vi "TDMS Close Retry.vi"(4 "Release File? (T)":bool=TRUE, 6 "New TDMS File Name (Optional)":string, 7 "TDMS Path":path, 8 "error in (no error)":errorcluster, 9 "Operation (0:open)":T1(ring)=enum."open (read-only)", 11 "TDMS File Ref":refnum<k34>) -> (0 "error out":errorcluster, 3 "TDMS Path Out":path, 5 "Execution Time (ms)":u32)   [LabVIEW 2011]
uses:
  Summitek EXT/OpenG EXT/file/file.llb/Convert File Extension (Path)__ogtk.vi
  Summitek EXT/OpenG EXT/file/file.llb/File Exists - Scalar__ogtk.vi
  Summitek EXT/OpenG EXT/file/file.llb/Strip Path Extension - Path__ogtk.vi
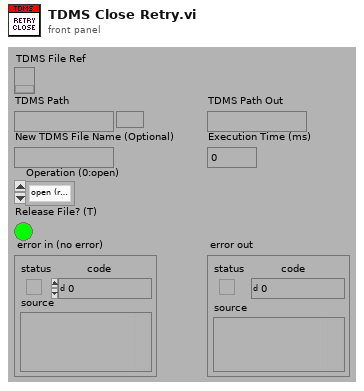
[diagram p1: front panel]
types:
  T1 = enum16{"open", "open or create", "create or replace", "create", "open (read-only)"}
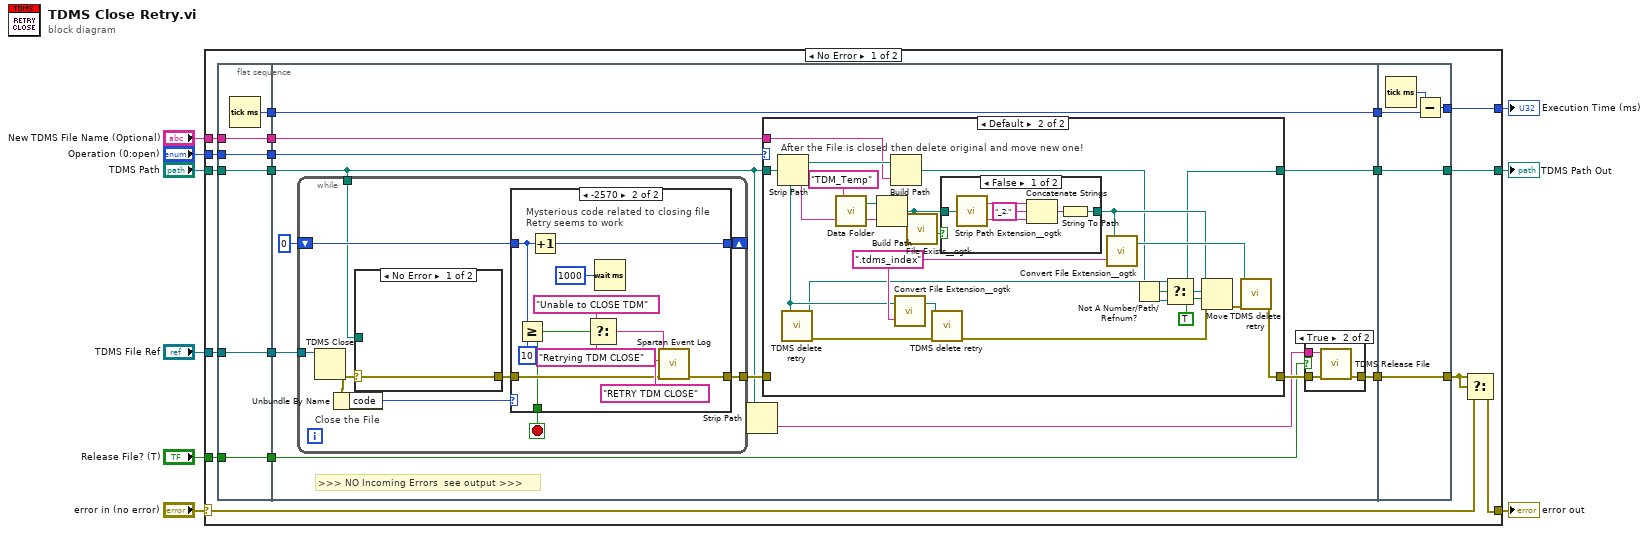
[diagram p0: block diagram]
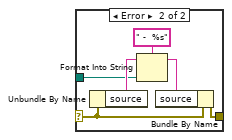
[diagram p5: hidden frame]
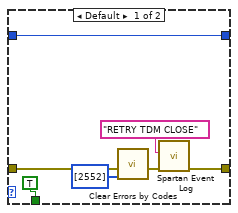
[diagram p6: hidden frame]
diagram:
  n1 = case shown="No Error" "error in (no error)" {
    selector: "error in (no error)" -> [w16 w121]
    tunnel: "TDMS File Ref" -> [w22 _]
    tunnel: "Operation (0:open)" -> [w21 _]
    tunnel: "TDMS Path" -> [w20 w120]
    tunnel: [w19 _] -> w6
    tunnel: [w18 w121] -> w5
    tunnel: [w15 w120] -> w3
    tunnel: "New TDMS File Name (Optional)" -> [w12 _]
    tunnel: "Release File? (T)" -> [w10 _]
    frame No Error {
      n2 = flat-sequence {
        tunnel: w20 -> [w32]
        tunnel: w21 -> [w33]
        tunnel: w22 -> [w34]
        tunnel: [w34] -> w28
        tunnel: [w33] -> w27
        tunnel: [w32] -> w26
        tunnel: [w31] -> w25
        tunnel: [w30] -> w13
        tunnel: w12 -> [w30]
        tunnel: [w29] -> w11
        tunnel: w10 -> [w29]
        tunnel: [w38] -> w24
        tunnel: w28 -> [w45]
        tunnel: w27 -> [w44]
        tunnel: w26 -> [w37]
        tunnel: [w42] -> w23
        tunnel: w25 -> [w42]
        tunnel: [w40] -> w14
        tunnel: w13 -> [w41]
        tunnel: w11 -> [w35]
        tunnel: [w119] -> w17
        tunnel: w24 -> [w119]
        tunnel: w23 -> [w117]
        tunnel: [w116] -> w19
        tunnel: [w115] -> w15
        tunnel: w14 -> [w115]
        frame #0 {
          n3 = Tick Count (ms)() -> (millisecond timer value=w31:u32)
        }
        frame #1 {
          # ">>> NO Incoming Errors  see output >>>"
          n4 = while {
            tunnel: w45 -> [w89]
            shift-right: [w85] -> _
            shift-left: 0 -> [w86]
            tunnel: [w84] -> w43
            tunnel: w37 -> [w81]
            stop <- w88 stop-if-true
            # "Close the File"
            n5 = TDMS Close(11:w89) -> (0:w82:errorcluster)  [unwired: 1 in, 1 out]
            n6 = Unbundle By Name(w82) -> ("code"=w87:i32)
            n7 = case shown="No Error" w82 {
              selector: w82 -> [w90 w93]
              tunnel: w81 -> [_ w94]
              tunnel: [w90 w91] -> w83
              frame No Error {
              }
              frame Error {
                n8 = Unbundle By Name(w93) -> ("source"=w95:string)
                n9 = Format Into String(format string=" -  %s", initial string=w95, w94) -> (resulting string=w92:string)  [unwired: 1 in, 1 out]
                n10 = Bundle By Name(cluster=w93, "source"=w92) -> (w91:errorcluster)
              }
            }
            n11 = case shown="-2570" w87 {
              tunnel: [TRUE ("T button?") w106] -> w88
              tunnel: w83 -> [w98 w113]
              tunnel: w86 -> [w102 w111]
              tunnel: [w102 w112] -> w85
              tunnel: [w101 w105] -> w84
              frame Default {
                n12 = call "Clear Errors by Codes.vi"("Error Codes\nto Clear (Empty)"=i32[] [2552] ("Error Codes\nto Clear (Empty)"), "error in (no error)"=w98) -> ("error out"=w97:errorcluster)  [unwired: 5 out]
                n13 = call "Spartan Event Log.vi"("error in (no error)"=w97, "module (\"\")"="RETRY TDM CLOSE") -> ("error out"=w101:errorcluster)  [unwired: 6 in]
              }
              frame -2570 {
                # "Mysterious code related to closing file\nRetry seems to work"
                n14 = Greater Or Equal?(x=w111, y=10) -> (x >= y?=w106:bool)
                n15 = Increment(x=w111) -> (x+1=w112:i32)
                n16 = Select(t="Unable to CLOSE TDM" ("message (\"\")"), s=w106, f="Retrying TDM CLOSE" ("message (\"\")")) -> (s? t:f=w107:string)
                n17 = Wait (ms)(milliseconds to wait=u32 1000) -> ()  [unwired: 1 out]
                n18 = call "Spartan Event Log.vi"("error in (no error)"=w113, "module (\"\")"="RETRY TDM CLOSE", "message (\"\")"=w107) -> ("error out"=w105:errorcluster)  [unwired: 5 in]
              }
            }
          }
          n19 = Strip Path(path=w37) -> (name=w36:string)  [unwired: 1 out]
          n20 = case shown="Default" w44 {
            tunnel: [w52 w70] -> w39
            tunnel: w43 -> [w52 _]
            tunnel: w37 -> [w51 w60]
            tunnel: w41 -> [_ w58]
            tunnel: [w51 w54] -> w40
            frame "create or replace", "open (read-only)" {
              # "The query TDM use the \"create or replace\" mode for the files.\nThey aren't in the search area.\nRead only operations shouldn't be affected either"
            }
            frame Default {
              w61 = ".tdms_index" ("regular expression")
              # "After the File is closed then delete original and move new one!"
              n21 = Strip Path(path=w60) -> (stripped path=w59:path, name=w73:string)
              n22 = call "TDMS delete retry.vi"("path (use dialog)"=w60) -> ("error out"=w68:errorcluster, "deleted path"=w56:path)  [unwired: 9 out]
              n23 = call "Data Folder.vi"("Relative Path (\"\" - Folder)"="TDM_Temp" ("Relative Path (\"\" - Folder)")) -> ("Data Folder"=w72:path)  [unwired: 2 in]
              n24 = Build Path(base path=w72, name or relative path=w73) -> (appended path=w63:path)
              n25 = Build Path(base path=w59, name or relative path=w58) -> (appended path=w55:path)
              n26 = call-poly "Convert File Extension__ogtk.vi"("new ending (none)"=w61, "file name"=w60) -> ("new filename"=w67:path)  [unwired: 1 out]
              n27 = call-poly "File Exists__ogtk.vi"("file path"=w63) -> ("exists"=w64:bool)  [unwired: 6 in, 1 out]
              n28 = call "TDMS delete retry.vi"("error in"=w68, "path (use dialog)"=w67) -> ("error out"=w71:errorcluster)  [unwired: 9 out]
              n29 = case shown="False" w64 {
                tunnel: w63 -> [w74 w80]
                tunnel: [w75 w80] -> w62
                frame False {
                  n30 = call-poly "Strip Path Extension__ogtk.vi"("path"=w74) -> ("root"=w77:string, "extension"=w76:string)
                  n31 = Concatenate Strings(w77, "_2." ("string"), w76) -> (w79:string)
                  n32 = String To Path(string=w79) -> (path=w75:path)
                }
                frame True {
                }
              }
              n33 = call-poly "Convert File Extension__ogtk.vi"("new ending (none)"=w61, "file name"=w62) -> ("new filename"=w69:path)  [unwired: 1 out]
              n34 = Not A Number/Path/Refnum?(number/path/refnum=w55) -> (NaN/Path/Refnum?=w57:bool)
              n35 = Select(t=w56, s=w57, f=w55) -> (s? t:f=w54:path)
              n36 = Move(source path=w62, error in=w71, 9:TRUE ("overwrite (F)"), 10:w54) -> (error out=w65:errorcluster)  [unwired: 3 out]
              n37 = call "TDMS delete retry.vi"("error in"=w65, "path (use dialog)"=w69) -> ("error out"=w70:errorcluster)  [unwired: 9 out]
            }
          }
          n38 = case shown="True" w35 {
            tunnel: w39 -> [w47 w50]
            tunnel: [w47 w49] -> w38
            tunnel: w36 -> [_ w48]
            frame False {
            }
            frame True {
              n39 = call "TDMS Release File.vi"("error in (no error)"=w50, "Filename"=w48) -> ("error out"=w49:errorcluster)  [unwired: 9 in]
            }
          }
        }
        frame #2 {
          n40 = Tick Count (ms)() -> (millisecond timer value=w118:u32)
          n41 = Subtract(x=w118, y=w117) -> (x-y=w116:u32)
        }
      }
      n42 = Select(t=w17, s=w17, f=w16) -> (s? t:f=w18:errorcluster)
    }
    frame Error {
    }
  }
  "error out" <- w5
  "Execution Time (ms)" <- w6
  "TDMS Path Out" <- w3
